vi "SECADO_calculos.vi"(7 "dt.ciclo, s":dbl format="%.1f", 8 "error in (no error)":errorcluster, 9 "datos.Ensayo.in":T1 {"Temp.termopar.9, C" format="%.2f"; "Temp.termopar.8, C" format="%.2f"; "Temp.termopar.7, C" format="%.2f"; "Porosidad," format="%.2f"; "Vel.air.reactor, m/s" format="%.2f"; "Q.evaporacion, W" format="%.2f"; "Q.aire.seco, W" format="%.2f"; "Humedad.lecho, f1" format="%.2f"; "Temperatura.ext, C" format="%.2f"; "Humedad.Rel.ext, f1" format="%.2f"; "Q.set.caudal, g/s" format="%.2f"; "Temp.termopar.6, C" format="%.2f"; "Temp.termopar.5, C" format="%.2f"; "P116.output, W" format="%.2f"; "Agua.evapor, g/s" format="%.2f"; "Humedad.rel.3, f1" format="%.2f"; "Temp.pt100.4, C" format="%.2f"; "Temp.pt100.3, C" format="%.2f"; "Q.caudal, g/s" format="%.2f"; "Humedad.rel.4, f1" format="%.2f"; "P116.temperatura, C" format="%.2f"; "P116.set.temp, C" format="%.2f"; "P116.output, %" format="%.2f"; "Temp.pt100.2, C" format="%.2f"; "Presion.dif, Pa" format="%.2f"; "Temp.pt100.1, C" format="%.2f"; "Tiempo (min)" format="%.2f"}, 10 "Constantes.Ensayo":T3={"Num.Ensayo"=0, "Diam_reactor, cm"=1.0, "Resistencia, ohm"=50.0, "Voltaje_resist, vac"=230.0, "Hum_ext, f1"=60.0, "Vel.min_fluido, m/s"=1.0, "Vel_arrastre, m/s"=10.0, "SET Caudal_vent, g/s"=5.0} {"Vel_arrastre, m/s" format="%.2f"; "SET Caudal_vent, g/s" format="%.2f"; "Diam_reactor, cm" format="%.2f"; "Resistencia, ohm" format="%.2f"; "Voltaje_resist, vac" format="%.2f"; "Hum_ext, f1" format="%.2f"; "Vel.min_fluido, m/s" format="%.2f"}, 11 "Datos.Lecho":T2={"Clasificacion"="Grueso (2,5<Dp<4", "Masa, g"=500.0, "Altura, cm"=45.0, "Diam_part, mm"=5.0, "Dens_part, g/cm3"=1.0, "Hum_ini, f1"=60.0, "Temp_ini, C"=25.0} {"Hum_ini, f1" format="%.2f"; "Temp_ini, C" format="%.2f"; "Masa, g" format="%.2f"; "Altura, cm" format="%.2f"; "Diam_part, mm" format="%.2f"; "Dens_part, g/cm3" format="%.2f"}) -> (0 "error out":errorcluster, 1 "datos.Ensayo.out":T1 {"Temp.termopar.9, C" format="%.2f"; "Temp.termopar.8, C" format="%.2f"; "Temp.termopar.7, C" format="%.2f"; "Porosidad," format="%.2f"; "Vel.air.reactor, m/s" format="%.2f"; "Q.evaporacion, W" format="%.2f"; "Q.aire.seco, W" format="%.2f"; "Humedad.lecho, f1" format="%.2f"; "Temperatura.ext, C" format="%.2f"; "Humedad.Rel.ext, f1" format="%.2f"; "Q.set.caudal, g/s" format="%.2f"; "Temp.termopar.6, C" format="%.2f"; "Temp.termopar.5, C" format="%.2f"; "P116.output, W" format="%.2f"; "Agua.evapor, g/s" format="%.2f"; "Humedad.rel.3, f1" format="%.2f"; "Temp.pt100.4, C" format="%.2f"; "Temp.pt100.3, C" format="%.2f"; "Q.caudal, g/s" format="%.2f"; "Humedad.rel.4, f1" format="%.2f"; "P116.temperatura, C" format="%.2f"; "P116.set.temp, C" format="%.2f"; "P116.output, %" format="%.2f"; "Temp.pt100.2, C" format="%.2f"; "Presion.dif, Pa" format="%.2f"; "Temp.pt100.1, C" format="%.2f"; "Tiempo (min)" format="%.2f"})   [LabVIEW 2017]
uses:
  Typedefs/SECADO_datos.Ensayo--Cluster.ctl
  Typedefs/SECADO_constantes.Ensayo--Cluster.ctl
  Typedefs/SECADO_datos.Lecho--Cluster.ctl
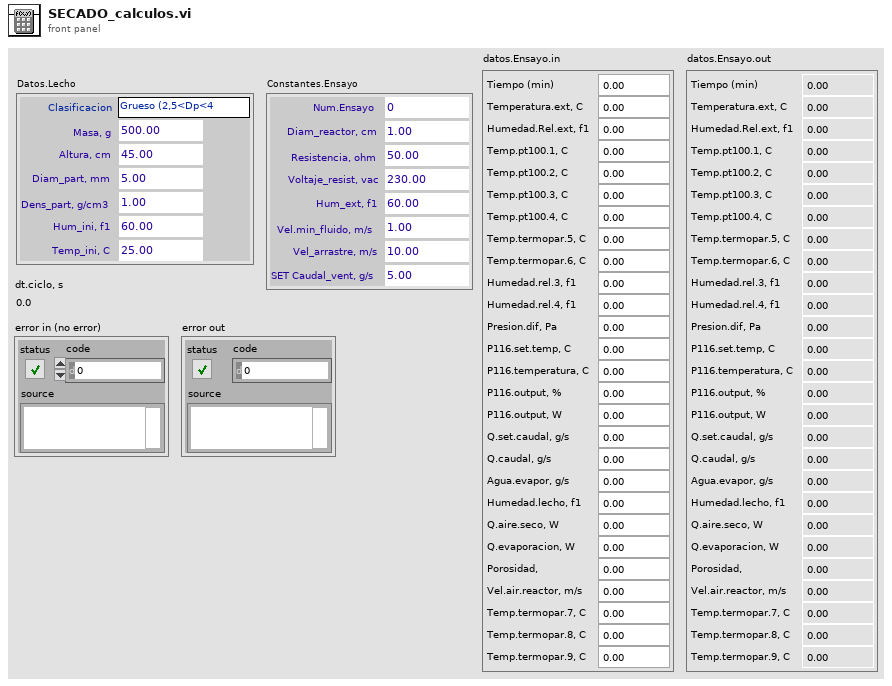
[diagram p1: front panel]
types:
  T1 = typedef "SECADO_datos.Ensayo--Cluster.ctl" = cluster{"Tiempo (min)":dbl, "Temperatura.ext, C":dbl, "Humedad.Rel.ext, f1":dbl, "Temp.pt100.1, C":dbl, "Temp.pt100.2, C":dbl, "Temp.pt100.3, C":dbl, "Temp.pt100.4, C":dbl, "Temp.termopar.5, C":dbl, "Temp.termopar.6, C":dbl, "Humedad.rel.3, f1":dbl, "Humedad.rel.4, f1":dbl, "Presion.dif, Pa":dbl, "P116.set.temp, C":dbl, "P116.temperatura, C":dbl, "P116.output, %":dbl, "P116.output, W":dbl, "Q.set.caudal, g/s":dbl, "Q.caudal, g/s":dbl, "Agua.evapor, g/s":dbl, "Humedad.lecho, f1":dbl, "Q.aire.seco, W":dbl, "Q.evaporacion, W":dbl, "Porosidad, ":dbl, "Vel.air.reactor, m/s":dbl, "Temp.termopar.7, C":dbl, "Temp.termopar.8, C":dbl, "Temp.termopar.9, C":dbl}
  T2 = typedef "SECADO_datos.Lecho--Cluster.ctl" = cluster{"Clasificacion":string, "Masa, g":dbl, "Altura, cm":dbl, "Diam_part, mm":dbl, "Dens_part, g/cm3":dbl, "Hum_ini, f1":dbl, "Temp_ini, C":dbl}
  T3 = typedef "SECADO_constantes.Ensayo--Cluster.ctl" = cluster{"Num.Ensayo":i32, "Diam_reactor, cm":dbl, "Resistencia, ohm":dbl, "Voltaje_resist, vac":dbl, "Hum_ext, f1":dbl, "Vel.min_fluido, m/s":dbl, "Vel_arrastre, m/s":dbl, "SET Caudal_vent, g/s":dbl}
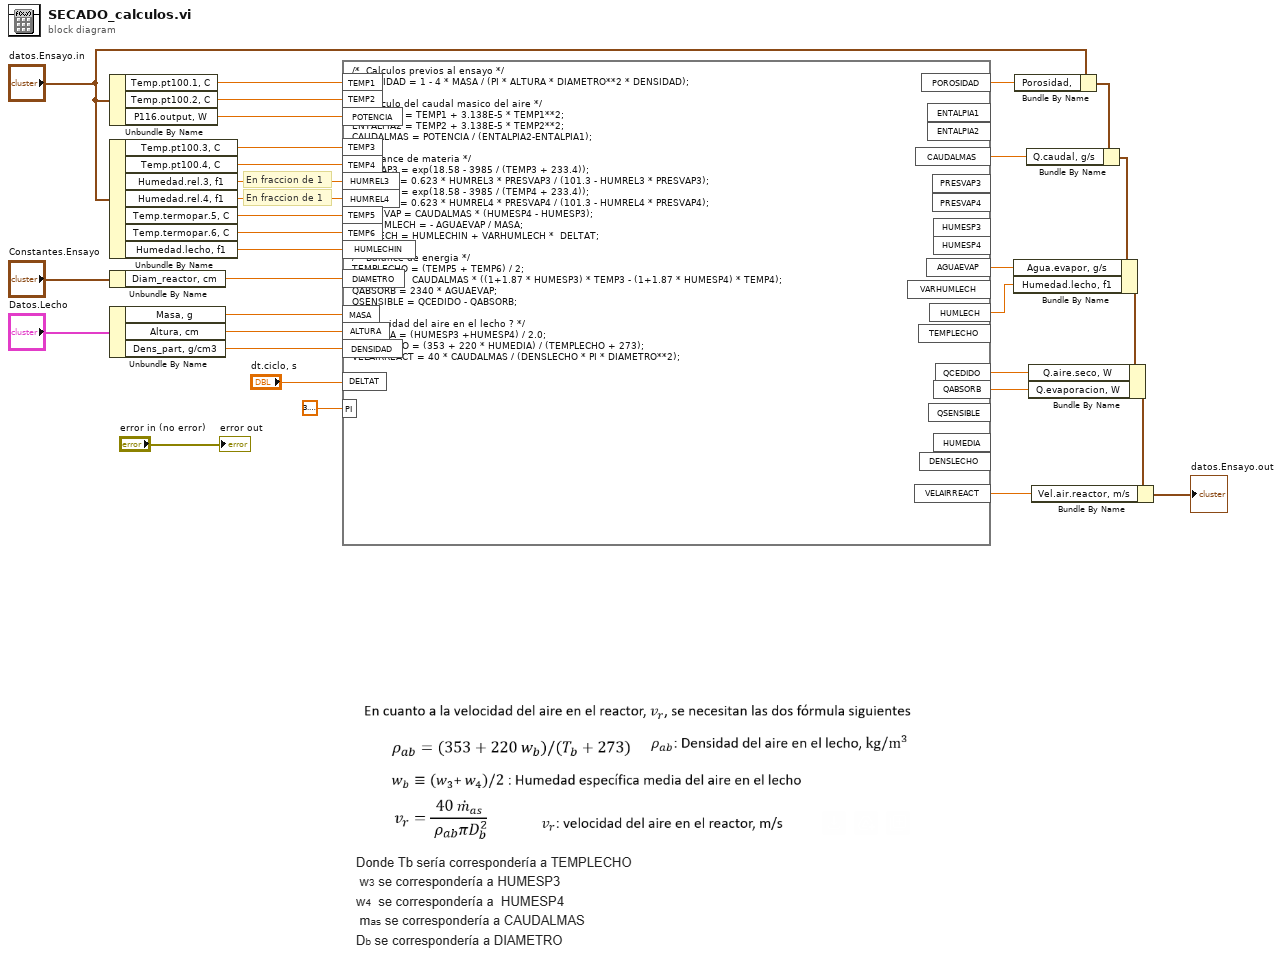
[diagram p0: block diagram]
diagram:
  # "En fraccion de 1"
  # "En fraccion de 1"
  n1 = Unbundle By Name("datos.Ensayo.in") -> ("Temp.pt100.1, C"=w23:dbl, "Temp.pt100.2, C"=w22:dbl, "P116.output, W"=w21:dbl)
  n2 = Unbundle By Name("datos.Ensayo.in") -> ("Temp.pt100.3, C"=w16:dbl, "Temp.pt100.4, C"=w15:dbl, "Humedad.rel.3, f1"=w14:dbl, "Humedad.rel.4, f1"=w13:dbl, "Temp.termopar.5, C"=w11:dbl, "Temp.termopar.6, C"=w10:dbl, "Humedad.lecho, f1"=w5:dbl)
  n3 = Unbundle By Name("Constantes.Ensayo") -> ("Diam_reactor, cm"=w26:dbl)
  n4 = Unbundle By Name("Datos.Lecho") -> ("Masa, g"=w28:dbl, "Altura, cm"=w27:dbl, "Dens_part, g/cm3"=w25:dbl)
  n5 = formula code="/*  Calculos previos al ensayo */\nPOROSIDAD = 1 - 4 * MASA / (PI * ALTURA * DIAMETRO**2 * DENSIDAD);\n\n/*  Calculo del caudal masico del aire */\nENTALPIA1 = TEMP1 + 3.138E-5 * TEMP1**2;\nENTALPIA2 = TEMP2 + 3.138E-5 * TEMP2**2;\nCAUDALMAS = POTENCIA / (ENTALPIA2-ENTALPIA1);\n\n/*  Balance de materia */\nPRESVAP3 = exp(18.58 - 3985 / (TEMP3 + 233.4));\nHUMESP3 = 0.623 * HUMREL3 * PRESVAP3 / (101.3 - HUMREL3 * PRESVAP3);\nPRESVAP4 = exp(18.58 - 3985 / (TEMP4 + 233.4));\nHUMESP4 = 0.623 * HUMREL4 * PRESVAP4 / (101.3 - HUMREL4 * PRESVAP4);\nAGUAEVAP = CAUDALMAS * (HUMESP4 - HUMESP3);  \nVARHUMLECH = - AGUAEVAP / MASA;\nHUMLECH = HUMLECHIN + VARHUMLECH *  DELTAT;\n\n/*  Balance de energia */\nTEMPLECHO = (TEMP5 + TEMP6) / 2;\nQCEDIDO =  CAUDALMAS * ((1+1.87 * HUMESP3) * TEMP3 - (1+1.87 * HUMESP4) * TEMP4);\nQABSORB = 2340 * AGUAEVAP;\nQSENSIBLE = QCEDIDO - QABSORB;\n \n/* Velocidad del aire en el lecho ? */\nHUMEDIA = (HUMESP3 +HUMESP4) / 2.0;\nDENSLECHO = (353 + 220 * HUMEDIA) / (TEMPLECHO + 273);\nVELAIRREACT = 40 * CAUDALMAS / (DENSLECHO * PI * DIAMETRO**2);"("MASA"=w28, "ALTURA"=w27, "DIAMETRO"=w26, "DENSIDAD"=w25, "PI"=3.141592653589793, "TEMP1"=w23, "TEMP2"=w22, "POTENCIA"=w21, "TEMP3"=w16, "TEMP4"=w15, "HUMREL3"=w14, "HUMREL4"=w13, "TEMP5"=w11, "TEMP6"=w10, "HUMLECHIN"=w5, "DELTAT"="dt.ciclo, s") -> ("POROSIDAD"=w18:dbl, "CAUDALMAS"=w20:dbl, "AGUAEVAP"=w12:dbl, "HUMLECH"=w9:dbl, "QCEDIDO"=w8:dbl, "QABSORB"=w7:dbl, "VELAIRREACT"=w1:dbl)  [unwired: 11 out]
  n6 = Bundle By Name(cluster="datos.Ensayo.in", "Porosidad,"=w18) -> (w19:T1)
  n7 = Bundle By Name(cluster=w19, "Q.caudal, g/s"=w20) -> (w32:T1)
  n8 = Bundle By Name(cluster=w32, "Agua.evapor, g/s"=w12, "Humedad.lecho, f1"=w9) -> (w6:T1)
  n9 = Bundle By Name(cluster=w6, "Q.aire.seco, W"=w8, "Q.evaporacion, W"=w7) -> (w3:T1)
  n10 = Bundle By Name(cluster=w3, "Vel.air.reactor, m/s"=w1) -> (→"datos.Ensayo.out":T1)
  "error out" <- "error in (no error)"
